vi "KG get mw sp.vi"(8 "Fehler (Eingang, kein Fehler)":errorcluster, 10 "pump":u32, 11 "VISA-Ressourcenname":refnum<visa-resource-name>) -> (0 "Fehler (Ausgang)":errorcluster, 1 "Kommando gesendet":string, 2 "Flow":dbl, 3 "VISA-Ressourcenname (Ausgang)":refnum<visa-resource-name>)   [LabVIEW 2020, in "Linearisierung v2.lvlib" / "Gasteiler.lvlib" / "HovaCAL_Interface.lvlib" / "KGN.lvlib" / "get.lvlib"]
uses:
  get.lvlib
  KGN.lvlib
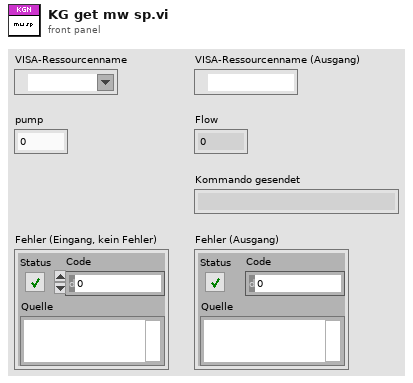
[diagram p1: front panel]
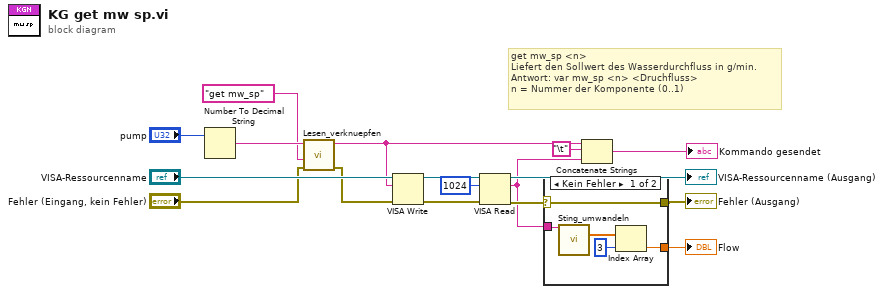
[diagram p0: block diagram]
diagram:
  # "get mw_sp <n>\nLiefert den Sollwert des Wasserdurchfluss in g/min.\nAntwort: var mw_sp <n> <Druchfluss>\nn = Nummer der Komponente (0..1)"
  n1 = Number To Decimal String(number="pump") -> (decimal integer string=w8:string)  [unwired: 1 in]
  n2 = call "Lesen_verknuepfen.vi"("error in (no error)"="Fehler (Eingang, kein Fehler)", "Order"="get mw_sp" ("Schreibpuffer"), "param"=w8) -> ("error out"=w10:errorcluster, "Verknüpfter String"=w9:string)  [unwired: 7 in]
  n3 = VISA Write(VISA resource name="VISA-Ressourcenname", write buffer=w9, error in (no error)=w10) -> (VISA resource name out=w17:refnum<visa-resource-name>, error out=w16:errorcluster)  [unwired: 1 out]
  n4 = VISA Read(VISA resource name=w17, byte count=u32 1024 ("Byte-Anzahl"), error in (no error)=w16) -> (VISA resource name out=→"VISA-Ressourcenname (Ausgang)":refnum<visa-resource-name>, read buffer=w2:string, error out=w6:errorcluster)  [unwired: 1 out]
  n5 = case shown="Kein Fehler" w6 {
    selector: w6 -> [w21 _]
    tunnel: w2 -> [w22 _]
    tunnel: [w18 _] -> w4
    tunnel: [w21 _] -> w5
    frame No Error {
      n6 = call "Sting_umwandeln.vi"("Lesepuffer"=w22) -> ("Zahl array"=w19:dbl[])  [unwired: 8 in, 6 out]
      n7 = Index Array(array=w19, index=3 ("Index")) -> (element=w18:dbl)
    }
    frame Error {
    }
  }
  "Fehler (Ausgang)" <- w5
  "Flow" <- w4
  n8 = Concatenate Strings(w9, "\t", w2) -> (→"Kommando gesendet":string)
